vi "test recup periph.vi"() -> ()   [LabVIEW 2017]
panel:
  in  "Menu déroulant":u16(ring)
  out "Tableau 2":string[](array[string])
  out "Tableau":string[](array[string])
  out "standard output":string
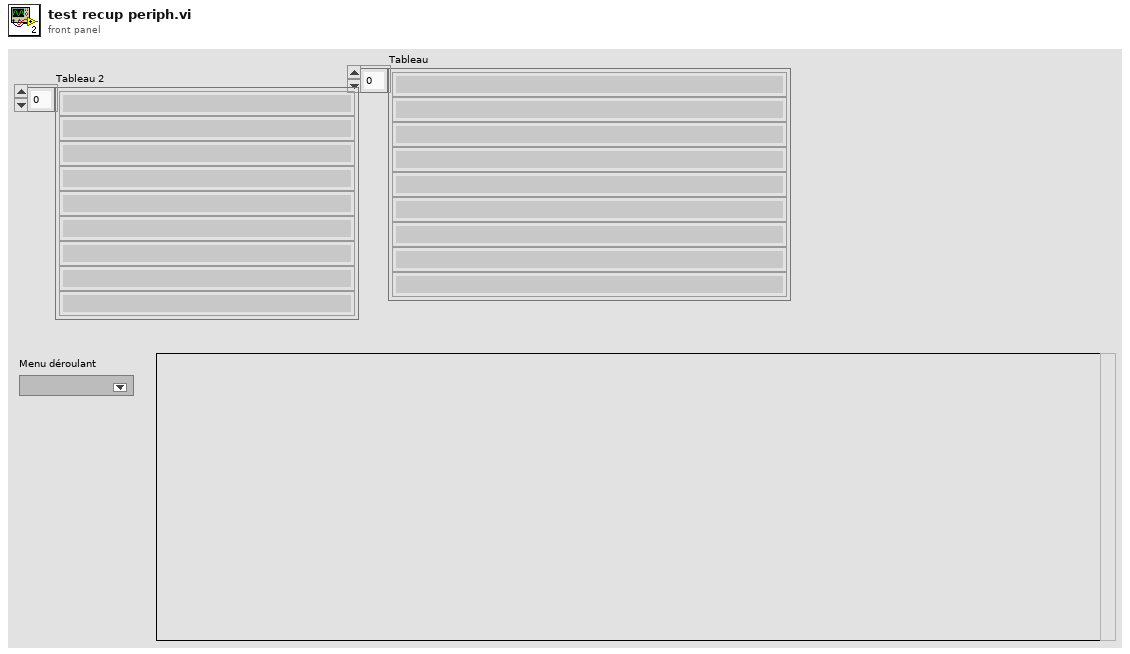
[diagram p1: front panel]
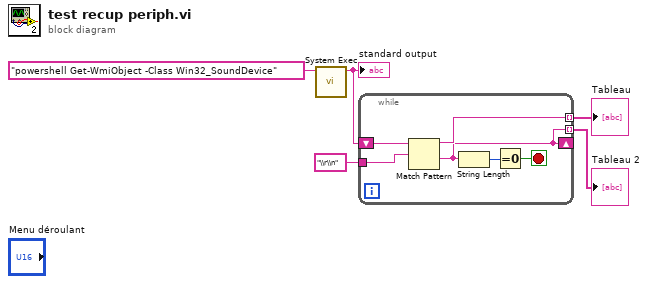
[diagram p0: block diagram]
diagram:
  n1 = call <vilib>:"System Exec.vi"("command line"="powershell Get-WmiObject -Class Win32_SoundDevice" ("name or relative path")) -> ("standard output"=w1:string)  [unwired: 7 in, 3 out]
  "standard output" <- w1
  n2 = while {
    tunnel: [w8] -> w4 mode=indexing
    shift-right: [w6] -> _
    shift-left: w1 -> [w9]
    tunnel: "\\r\\n" -> [w7]
    tunnel: [w6] -> w3 mode=indexing
    stop <- w10 stop-if-true
    n3 = Match Pattern(string=w9, regular expression=w7) -> (before substring=w8:string, after substring=w6:string)  [unwired: 1 in, 2 out]
    n4 = String Length(string=w6) -> (length=w11:i32)
    n5 = Equal To 0?(x=w11) -> (x = 0?=w10:bool)
  }
  "Tableau" <- w4
  "Tableau 2" <- w3
